vi "Benchmark Project.vi"() -> ()   [LabVIEW 2020]
doc: "This example gathers timing information about a VI's execution by running the VI over several iterations. The example obtains several consecutive timestamps, which are stored in an array and used to produce a histogram of execution time. The example can self-calibrate by subtracting out the overhead of calling NI Get Timestamp.vi from the array of timing data."
uses:
  <vilib>/Analysis/Matrix/Numeric/Conversions/Array To Matrix - RA.vi
  <vilib>/Analysis/Matrix/Numeric/Conversions/Array To Matrix - RA2.vi
  <vilib>/Analysis/Matrix/Numeric/Multiply/Multiply - RM,RM.vi
  <vilib>/NI_Real-Time Target Support.lvlib
  <vilib>/Analysis/Matrix/NI_Matrix.lvlib
panel:
  in  "vector size":i32=20
  out "Mean time (us)":dbl format="%.3g"
  out "Max jitter (us)":dbl format="%.3g"
  out "Standard deviation (us)":dbl format="%.3g"
  in  "Warmup iterations":i32=10
  in  "Calibrate?":bool
  in  "Iterations":i32=1000
  out "Execution histogram":T1(graph)
  out "Execution times (us)":dbl[](graph)
  # "Overview: Gathers timing information on VI execution by running it over several iterations.\nRequirements: LabVIEW Real-Time Module\nInstructions:\n1. In Measurement & Automation Explorer, ensure that LabVIEW Real-Time is installed on your RT target.  \n2. From the Project Explorer window, set the IP address of your RT target.\n3. From the front panel, select the number of iterations to run and the number of warmup iterations to exclude from the benchmark.\n4. Enable Calibrate? if you want to exclude the overhead of the timestamping operation.\n5. Open the block diagram and insert the code you want to benchmark in the #CodeNeeded section.\n6. Run the VI."
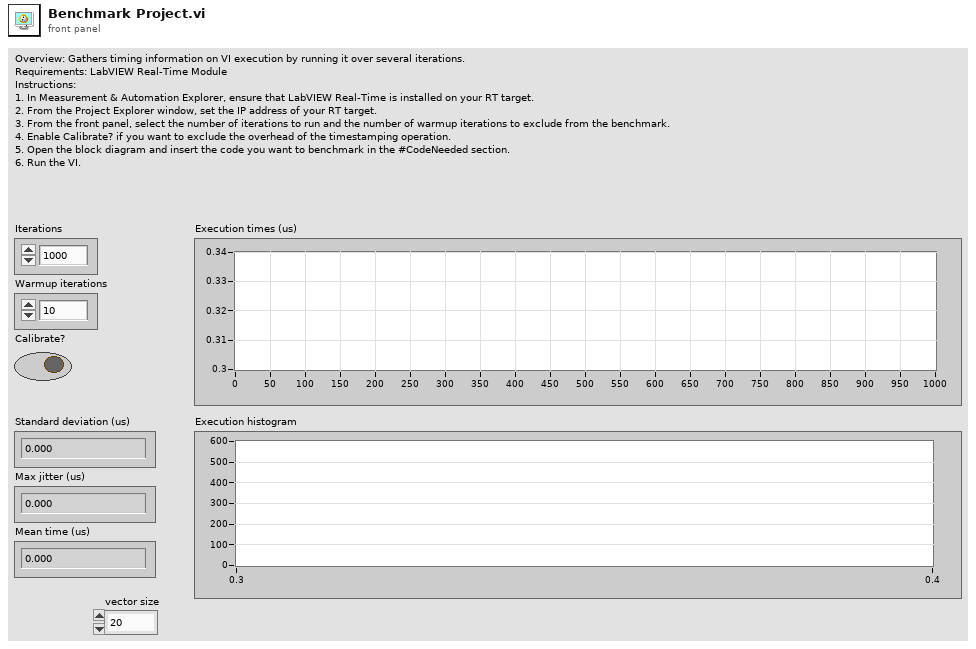
[diagram p1: front panel]
types:
  T1 = cluster{"X Values":dbl[], "Histogram: h(x)":i32[]}
  T2 = typedef "NI_Matrix.lvlib/RealMatrix.ctl" = dbl[][]
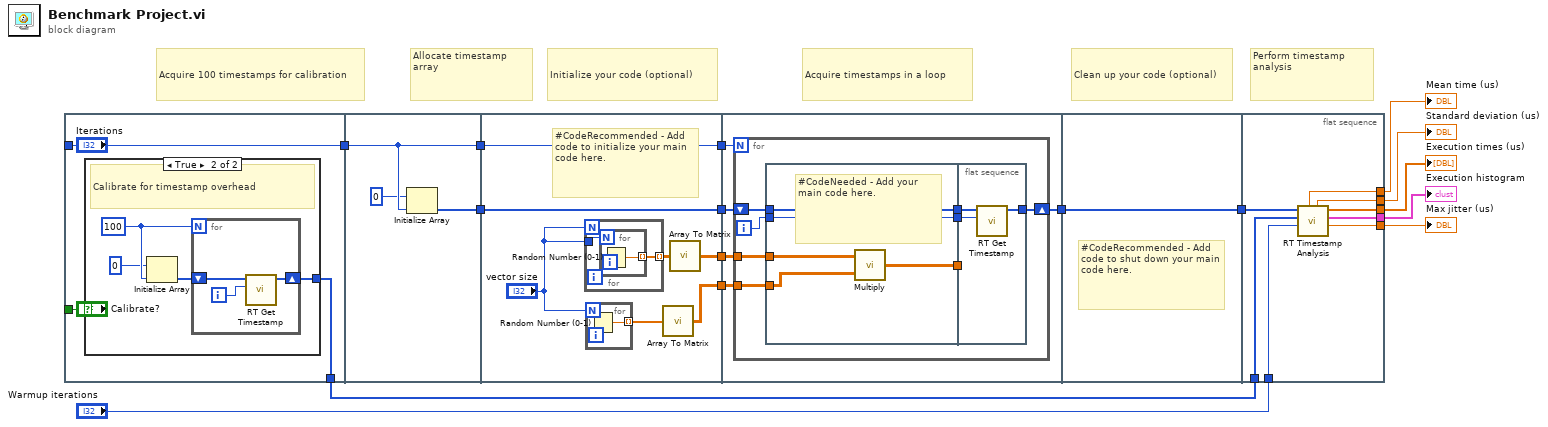
[diagram p0: block diagram]
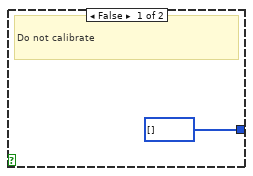
[diagram p2: hidden frame]
diagram:
  # "Perform timestamp analysis"
  # "Clean up your code (optional)"
  # "Acquire timestamps in a loop"
  # "Initialize your code (optional)"
  # "Allocate timestamp array"
  # "Acquire 100 timestamps for calibration"
  n1 = flat-sequence {
    tunnel: "Iterations" -> [w21]
    tunnel: [w21] -> w12
    tunnel: "Calibrate?" -> [w20]
    tunnel: [w19] -> w9
    tunnel: [w31] -> w14
    tunnel: [w32] -> w13
    tunnel: w12 -> [w31]
    tunnel: [w39] -> w16
    tunnel: [w38] -> w15
    tunnel: w14 -> [w39]
    tunnel: w13 -> [w38]
    tunnel: [w34] -> w2
    tunnel: [w33] -> w1
    tunnel: [w48] -> w17
    tunnel: w16 -> [w47]
    tunnel: w15 -> [w46]
    tunnel: w2 -> [w45]
    tunnel: w1 -> [w44]
    tunnel: w17 -> [w65]
    tunnel: [w65] -> w10
    tunnel: w10 -> [w73]
    tunnel: w9 -> [w72]
    tunnel: [w71] -> w3
    tunnel: [w70] -> w7
    tunnel: [w69] -> w6
    tunnel: [w68] -> w8
    tunnel: "Warmup iterations" -> [w67]
    tunnel: [w66] -> w4
    frame #0 {
      n2 = case shown="True" w20 {
        tunnel: [u64[] [] w26] -> w19
        frame False {
          # "Do not calibrate"
        }
        frame True {
          w24 = 100
          # "Calibrate for timestamp overhead"
          n3 = Initialize Array(u64 0, w24) -> (w25:u64[])
          n4 = for {
            N: w24 -> [_]
            shift-right: [w27] -> w26
            shift-left: w25 -> [w28]
            i -> [w29]
            n5 = call <vilib>:"RT Get Timestamp.vi"("iteration"=w29, "timestamp array in"=w28) -> ("timestamp array out"=w27:u64[])  [unwired: 1 in, 8 out]
          }
        }
      }
    }
    frame #1 {
      n6 = Initialize Array(u64 0, w31) -> (w32:u64[])
    }
    frame #2 {
      # "#CodeRecommended - Add code to initialize your main code here."
      n7 = for {
        N: "vector size" -> [_]
        tunnel: [w41] -> w36 mode=indexing
        tunnel: "vector size" -> [w40]
        n8 = for {
          N: w40 -> [_]
          tunnel: [w42] -> w41 mode=indexing
          n9 = Random Number (0-1)() -> (number: 0 to 1=w42:dbl)
        }
      }
      n10 = for {
        N: "vector size" -> [_]
        tunnel: [w43] -> w37 mode=indexing
        n11 = Random Number (0-1)() -> (number: 0 to 1=w43:dbl)
      }
      n12 = call-poly <vilib>:"Array To Matrix.vi"("Real 1D Array"=w37) -> ("Real Matrix (Column Vector)"=w33:T2)
      n13 = call-poly <vilib>:"Array To Matrix.vi"("Real 2D Array"=w36) -> ("Real Matrix"=w34:T2)
    }
    frame #3 {
      n14 = for {
        N: w47 -> [_]
        shift-right: [w56] -> w48
        shift-left: w46 -> [w55]
        tunnel: w45 -> [w51]
        tunnel: w44 -> [w50]
        i -> [w54]
        n15 = flat-sequence {
          tunnel: w55 -> [w61]
          tunnel: [w61] -> w53
          tunnel: w54 -> [w60]
          tunnel: [w60] -> w52
          tunnel: w51 -> [w59]
          tunnel: w50 -> [w58]
          tunnel: [w57] -> w49
          tunnel: [w64] -> w56
          tunnel: w53 -> [w62]
          tunnel: w52 -> [w63]
          tunnel: w49 -> [_]
          frame #0 {
            # "#CodeNeeded - Add your main code here."
            n16 = call-poly <vilib>:"Multiply.vi"("Real Matrix B"=w58, "Real Matrix A"=w59) -> ("A * B"=w57:T2)
          }
          frame #1 {
            n17 = call <vilib>:"RT Get Timestamp.vi"("iteration"=w63, "timestamp array in"=w62) -> ("timestamp array out"=w64:u64[])  [unwired: 1 in, 8 out]
          }
        }
      }
    }
    frame #4 {
      # "#CodeRecommended - Add code to shut down your main code here."
    }
    frame #5 {
      n18 = call <vilib>:"RT Timestamp Analysis.vi"("warmup iterations"=w67, "calibration array"=w72, "timestamp array"=w73) -> ("max jitter (uS)"=w70:dbl, "execution histogram"=w71:T1, "execution times (uS)"=w68:dbl[], "standard deviation (uS)"=w69:dbl, "mean time (uS)"=w66:dbl)  [unwired: 1 in, 3 out]
    }
  }
  "Execution times (us)" <- w8
  "Max jitter (us)" <- w7
  "Standard deviation (us)" <- w6
  "Execution histogram" <- w3
  "Mean time (us)" <- w4
